vi "Clear Buffers (No Objects).vi"(8 "error in (no error)":errorcluster, 11 "Cluster In":T10={"Channel Names"=[], "Channel Units"=[], "Most Recent Data Points"=[], "History Buffers"=[], "Ring Buffers"=[], "Exp Range Min"=0, "Exp Range Max"=0, "exposure mode"=enum."manual", "operation (meas. mode)"=enum."Measurement mode", "Exposure (ms)"=0, "Quiet Errors?"=FALSE, "Error Status"={"status"=FALSE, "code"=0, "source"=""}}) -> (0 "error out":errorcluster, 3 "Cluster Out":T10={"Channel Names"=[], "Channel Units"=[], "Most Recent Data Points"=[], "History Buffers"=[], "Ring Buffers"=[], "Exp Range Min"=0, "Exp Range Max"=0, "exposure mode"=enum."manual", "operation (meas. mode)"=enum."Measurement mode", "Exposure (ms)"=0, "Quiet Errors?"=FALSE, "Error Status"={"status"=FALSE, "code"=0, "source"=""}})   [LabVIEW 2009]
uses:
  Channel Names.ctl
  Channel Units.ctl
  Data Points.ctl
  Data Point.ctl
  Time.ctl
  X.ctl
  TX Graph.ctl
  Wavelength meter/HighFinesse WS5/Variable Typedefs.llb/Exposure Mode.ctl
  Wavelength meter/HighFinesse WS5/Control typedefs.llb/Measurement Mode.ctl
  Readable.lvclass
  Wavelength meter/HighFinesse WS5/HighFinesse WS5.lvlib
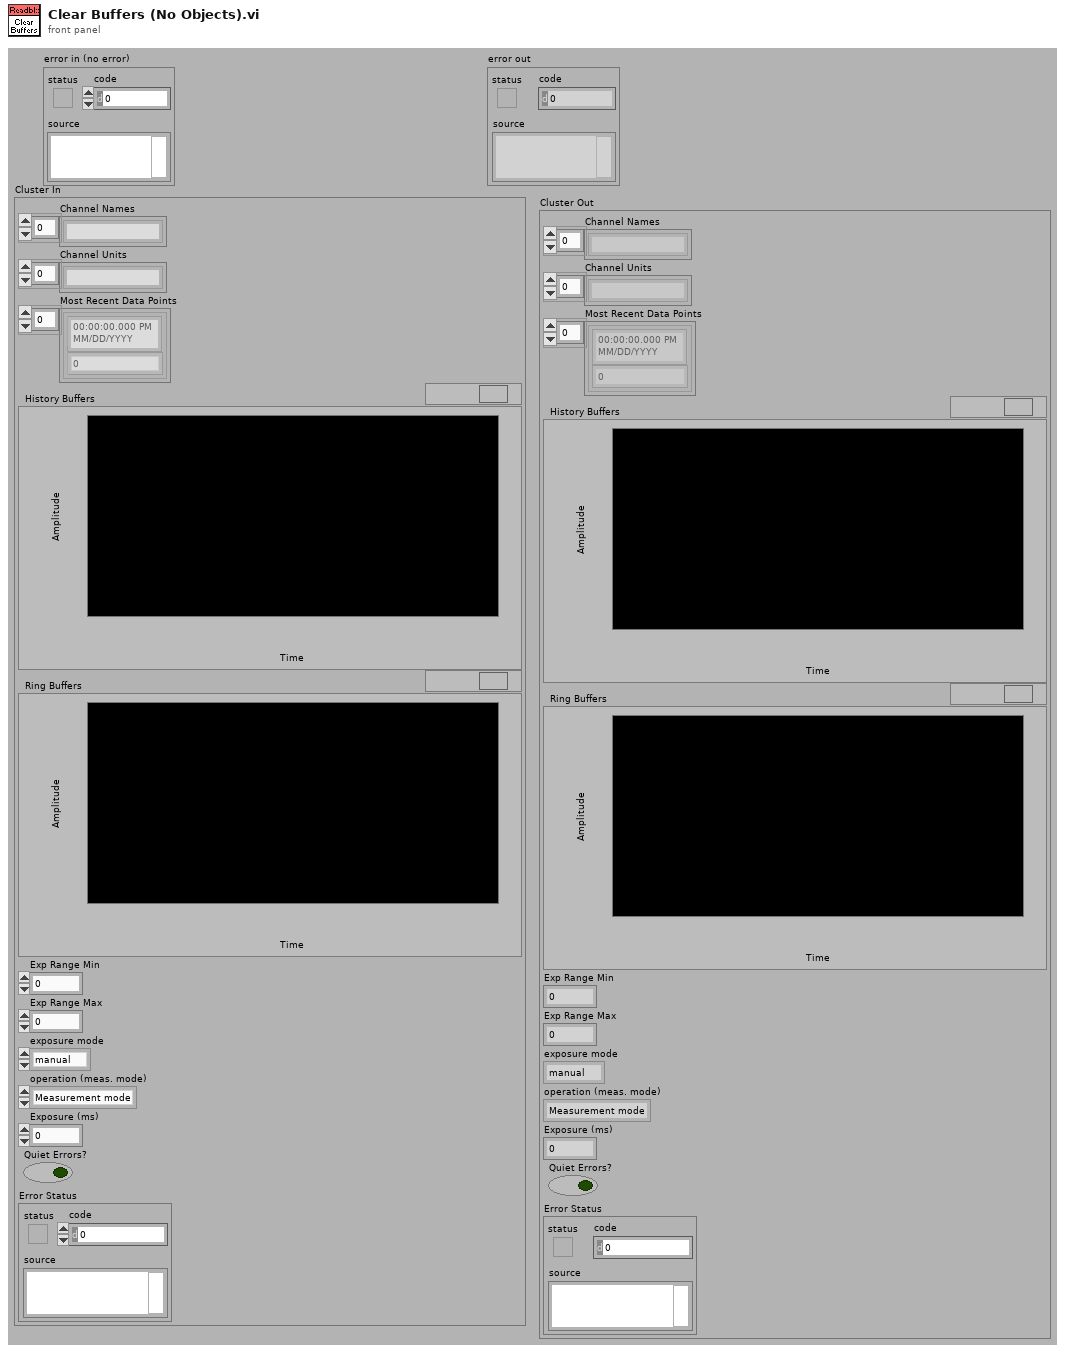
[diagram p1: front panel]
types:
  T1 = typedef "Readable.lvclass/Channel Names.ctl" = string[]
  T2 = typedef "Readable.lvclass/Channel Units.ctl" = string[]
  T3 = typedef "Readable.lvclass/Data Points.ctl" = T4[]
  T4 = typedef "Readable.lvclass/Data Point.ctl" = cluster{"t":T5, "x":T6}
  T5 = typedef "Readable.lvclass/Time.ctl" = timestamp
  T6 = typedef "Readable.lvclass/X.ctl" = dbl
  T7 = typedef "Readable.lvclass/TX Graph.ctl" = cluster{"Data Points":cluster{"t":timestamp, "x":dbl}[]}[]
  T8 = typedef "HighFinesse WS5.lvlib/Exposure Mode.ctl" = enum16{"manual", "automatic"}
  T9 = typedef "HighFinesse WS5.lvlib/Measurement Mode.ctl" = enum16{"Measurement off", "Adjustment mode", "Measurement mode"}
  T10 = cluster{"Channel Names":T1, "Channel Units":T2, "Most Recent Data Points":T3, "History Buffers":T7, "Ring Buffers":T7, "Exp Range Min":u32, "Exp Range Max":u32, "exposure mode":T8, "operation (meas. mode)":T9, "Exposure (ms)":u16, "Quiet Errors?":bool, "Error Status":errorcluster}
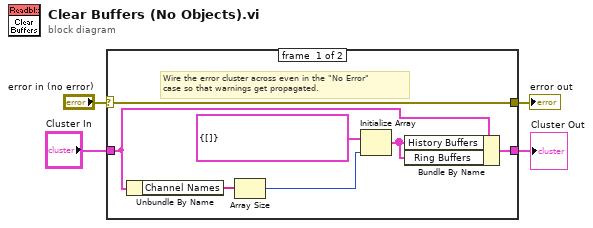
[diagram p0: block diagram]
diagram:
  n1 = case shown="No Error" "error in (no error)" {
    selector: "error in (no error)" -> [w11 w13]
    tunnel: [w11 w13] -> w3
    tunnel: [w9 w12] -> w1
    tunnel: "Cluster In" -> [w7 w12]
    frame #0 {
      # "Wire the error cluster across even in the \"No Error\"\ncase so that warnings get propagated."
      n2 = Unbundle By Name(w7) -> ("Channel Names"=w6:T1)
      n3 = Array Size(array=w6) -> (size(s)=w5:i32)
      n4 = Initialize Array(cluster{T4[]} {[]} ("output cluster"), w5) -> (w8:cluster{T4[]}[])
      n5 = Bundle By Name(cluster=w7, "History Buffers"=w8, "Ring Buffers"=w8) -> (w9:T10)
    }
    frame #1 {
    }
  }
  "error out" <- w3
  "Cluster Out" <- w1
